vi "Test - Thermal Chamber Controller_DQMH - Update Set Point 1-test_harness.vi"(11 "test case ID":string) -> (3 "result":bool)   [LabVIEW 2015]
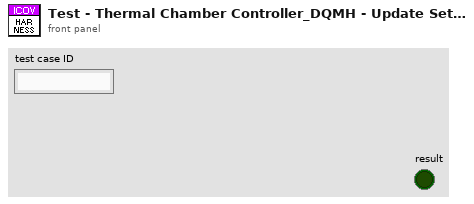
[diagram p1: front panel]
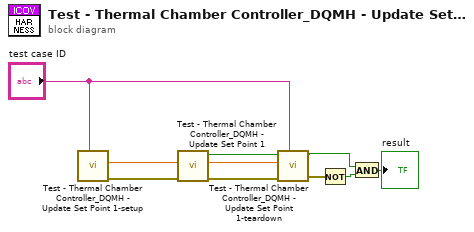
[diagram p0: block diagram]
diagram:
  n1 = call "Test - Thermal Chamber Controller_DQMH - Update Set Point 1-setup.vi"("test case ID"="test case ID") -> ("error out"=w8:errorcluster, "Temperature Set Point"=w9:dbl)  [unwired: 9 in]
  n2 = call "Test - Thermal Chamber Controller_DQMH - Update Set Point 1.vi"("error in (no error)"=w8, "Temperature Set Point Input"=w9) -> ("error out"=w7:errorcluster, "Temperature Set Point Result"=w6:dbl, "Success"=w5:bool)  [unwired: 7 in]
  n3 = call "Test - Thermal Chamber Controller_DQMH - Update Set Point 1-teardown.vi"("test case ID"="test case ID", "error in (no error)"=w7, "Temperature Set Point"=w6, "no error"=w5) -> ("error out"=w2:errorcluster, "result"=w3:bool)  [unwired: 6 in]
  n4 = Not(x=w2) -> (.not. x?=w4:bool)
  n5 = And(x=w3, y=w4) -> (x .and. y?=→"result":bool)
